vi "equipoSeleccionado.vi"(8 "error in (no error)":errorcluster, 11 "Dosimetro in":refnum<class "Dosimetro.lvclass">) -> (0 "error out":errorcluster, 2 "equipoSeleccionado":string, 3 "Dosimetro out":refnum<class "Dosimetro.lvclass">)   [LabVIEW 2019, in "Dosimetro.lvclass"]
uses:
  Dosimetro.lvclass
  Dosimetro.lvclass/Dosimetro.ctl
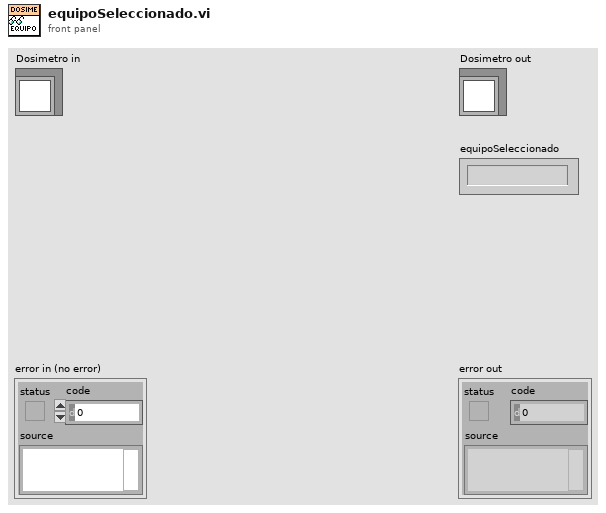
[diagram p1: front panel]
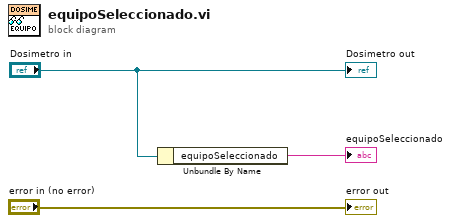
[diagram p0: block diagram]
diagram:
  n1 = Unbundle By Name("Dosimetro in") -> ("equipoSeleccionado"=→"equipoSeleccionado":string)
  "error out" <- "error in (no error)"
  "Dosimetro out" <- "Dosimetro in"
